vi "subvi_jenoptik_average_diff.vi"(1 "phase in":dbl[](array[numeric]) format="%.2f", 3 "window max":i32, 4 "window min":i32) -> (0 "Array":dbl[](array[numeric]) format="%.2f")   [LabVIEW 2019]
uses:
  <vilib>/Analysis/NI_AALPro.lvlib
  <vilib>/Analysis/NI_AALBase.lvlib
  <vilib>/Analysis/1siggen.llb/Ramp Pattern by Samples.vi
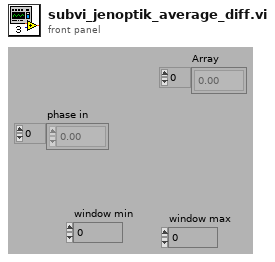
[diagram p1: front panel]
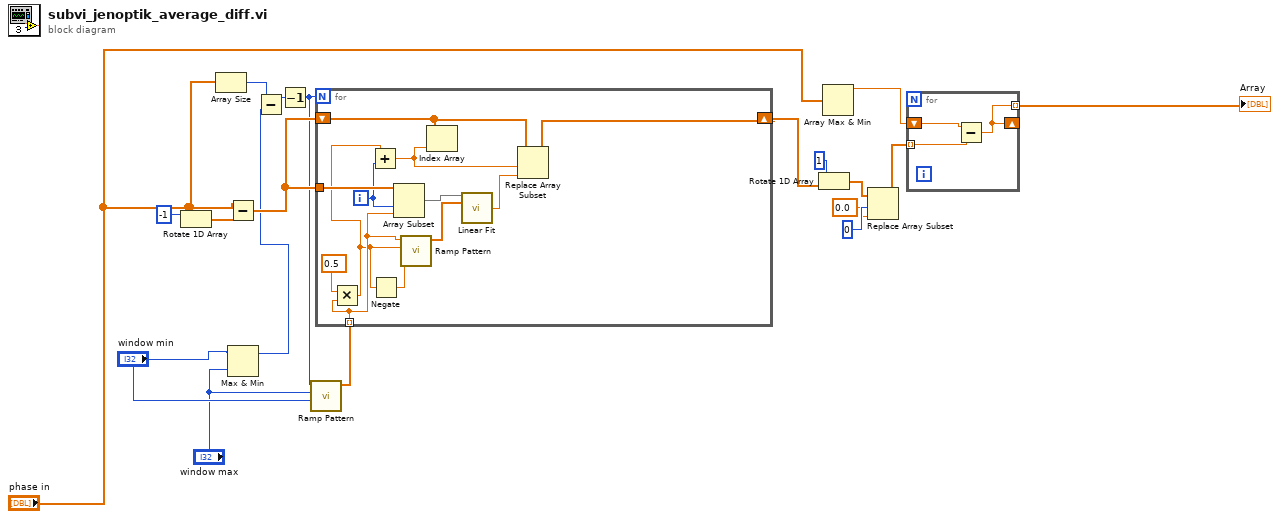
[diagram p0: block diagram]
diagram:
  n1 = Rotate 1D Array(1:"phase in", 2:i16 -1 ("n")) -> (0:w18:dbl[])
  n2 = Array Size(array="phase in") -> (size(s)=w11:i32)
  n3 = Subtract(x="phase in", y=w18) -> (x-y=w19:dbl[])
  n4 = Max & Min(x="window min", y="window max") -> (max(x,y)=w4:i32)  [unwired: 1 out]
  n5 = Subtract(x=w11, y=w4) -> (x-y=w12:i32)
  n6 = Decrement(x=w12) -> (x-1=w6:i32)
  n7 = call-poly <vilib>:"Ramp Pattern.vi"("start"="window min", "end"="window max", "samples"=w6) -> ("Ramp Pattern"=w5:dbl[])  [unwired: 7 in, 1 out]
  n8 = for {
    N: w6 -> [_]
    tunnel: w19 -> [w31]
    shift-right: [w27] -> w7
    shift-left: w19 -> [w28]
    tunnel: w5 -> [w25] mode=indexing
    i -> [w30]
    n9 = Multiply(x=0.5, y=w25) -> (x*y=w24:dbl)
    n10 = Add(x=w24, y=w30) -> (x+y=w29:dbl)
    n11 = Negate(x=w24) -> (-x=w23:dbl)
    n12 = Array Subset(array=w31, index=w30, length=w25) -> (w21:dbl[])
    n13 = call-poly <vilib>:"Ramp Pattern.vi"("start"=w23, "end"=w24, "samples"=w25) -> ("Ramp Pattern"=w22:dbl[])  [unwired: 7 in, 1 out]
    n14 = Index Array(array=w28, index=w29) -> ()  [unwired: 1 out]
    n15 = call <vilib>:"Linear Fit.vi"("Y"=w21, "X"=w22) -> ("intercept"=w20:dbl)  [unwired: 4 in, 9 out]
    n16 = Replace Array Subset(array=w28, new element=w20, index=w29) -> (w27:dbl[])
  }
  n17 = Rotate 1D Array(1:w7, 2:i16 1 ("n")) -> (0:w15:dbl[])
  n18 = Array Max & Min(array="phase in") -> (max value=w13:dbl)  [unwired: 3 out]
  n19 = Replace Array Subset(array=w15, new element=0.0 ("Element Data"), index=0 ("Index")) -> (w8:dbl[])
  n20 = for {
    tunnel: w8 -> [w34] mode=indexing
    shift-right: [w32] -> _
    shift-left: w13 -> [w33]
    tunnel: [w32] -> w1 mode=indexing
    n21 = Subtract(x=w33, y=w34) -> (x-y=w32:dbl)
  }
  "Array" <- w1
